vi "Save.vi"(7 "source paths":path[](array[path]), 8 "error in (no error)":errorcluster, 10 "processed sources":refnum<class "AB_Source.lvclass">[](array[class]), 11 "AB_EXE in":refnum<class "AB_EXE.lvclass">) -> (0 "error out":errorcluster, 1 "TypeInfo":string, 2 "source destination paths":path[](array[path]), 3 "AB_EXE out":refnum<class "AB_EXE.lvclass">, 4 "LEIFBuildData":u32, 5 "checksums":string[](array[string]))   [LabVIEW 2020, in "AB_EXE.lvclass"]
uses:
  <vilib>/AppBuilder/AB_Classes/EXE/AB_EXE.lvclass
  e:/builds/penguin/labview/branches/2020/dev/dist/vi.lib/AppBuilder/AB_Classes/TargetFile/AB_Targetfile.lvclass
  <vilib>/AppBuilder/AB_Classes/Source/AB_Source.lvclass
  <vilib>/AppBuilder/AB_Classes/Application/AB_Application.lvclass
  <vilib>/AppBuilder/AB_Classes/TargetFile/AB_Targetfile.lvclass
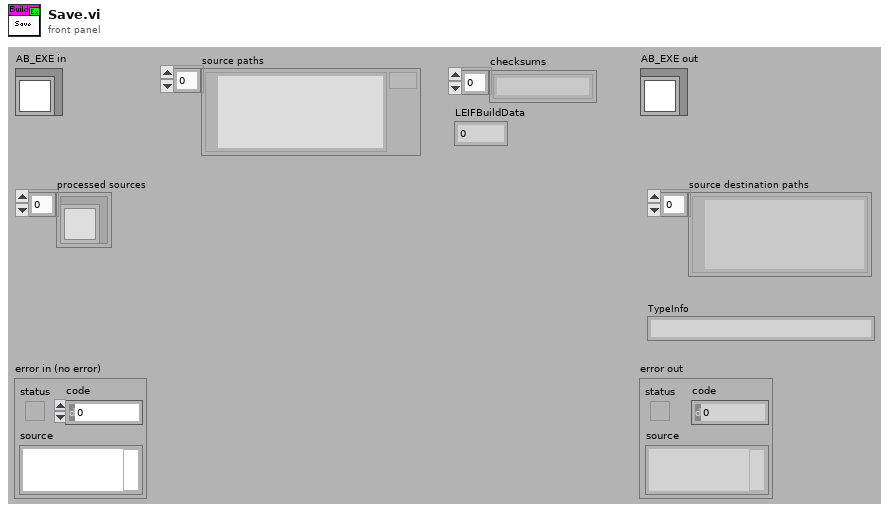
[diagram p1: front panel]
types:
  T1 = typedef "AB_Targetfile.ctl" = cluster{"targetfileName":string, "targetfileGUID":string, "enableDebugging":bool, "versionInfo":cluster{"productName":string, "legalCopyright":string, "companyName":string, "internalName":string, "fileDescription":string}, "eng_consolidatedTypeInfo":string, "fastFileFormat":bool, "eng_LEIFBuildData":u32, "versionIndependent":bool}
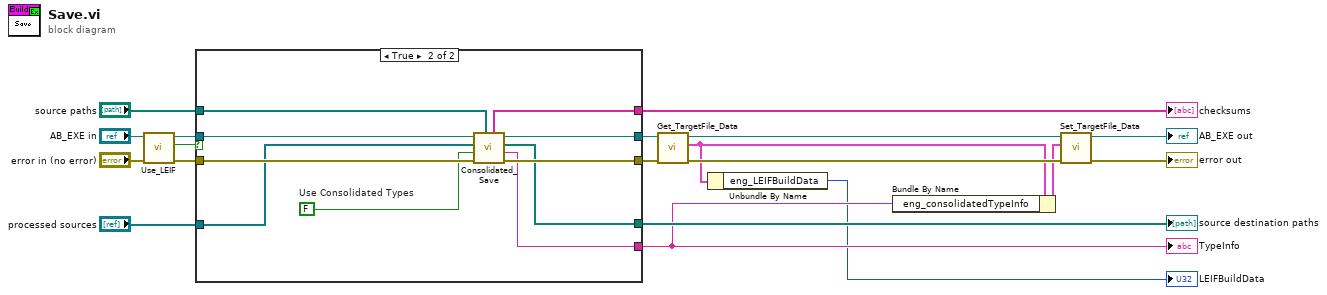
[diagram p0: block diagram]
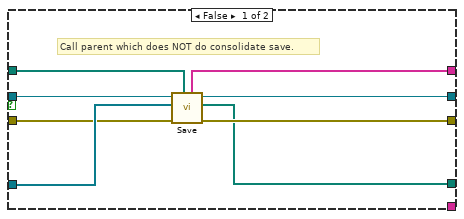
[diagram p2: hidden frame]
diagram:
  n1 = call <vilib>:"Use_LEIF.vi"("error in (no error)"="error in (no error)", "AB_Targetfile in"="AB_EXE in") -> ("error out"=w6:errorcluster, "use LEIF?"=w5:bool, "AB_Targetfile out"=w3:refnum<class "AB_EXE.lvclass">)  [unwired: 7 in]
  n2 = case shown="True" w5 {
    tunnel: "processed sources" -> [w23 w29]
    tunnel: w6 -> [w22 w30]
    tunnel: [w26 w36] -> w9
    tunnel: [w27 w35] -> w11
    tunnel: [_ w33] -> w8
    tunnel: "source paths" -> [w21 w31]
    tunnel: [w25 w34] -> w17
    tunnel: w3 -> [w24 w32]
    tunnel: [w20 w37] -> w16
    frame False {
      # "Call parent which does NOT do consolidate save."
      n3 = call-parent "Save.vi"("source paths"=w21, "error in"=w22, "processed sources"=w23, "AB_Build in"=w24) -> ("error out"=w26:errorcluster, "source destination paths"=w25:path[], "AB_Build out"=w27:refnum<class "AB_EXE.lvclass">, "checksums"=w20:string[])  [unwired: 2 in, 2 out]
    }
    frame True {
      w28 = FALSE  # Use Consolidated Types
      n4 = call <vilib>:"Consolidated_Save.vi"("source paths"=w31, "error in"=w30, "Use Consolidated Types"=w28, "processed sources"=w29, "AB_Targetfile in"=w32) -> ("error out"=w36:errorcluster, "TypeInfo"=w33:string, "source destination paths"=w34:path[], "AB_Targetfile out"=w35:refnum<class "AB_EXE.lvclass">, "checksums"=w37:string[])  [unwired: 2 in]
    }
  }
  "source destination paths" <- w17
  "TypeInfo" <- w8
  "checksums" <- w16
  n5 = call <vilib>:"Get_TargetFile_Data.vi"("error in (no error)"=w9, "AB_Targetfile in"=w11) -> ("error out"=w14:errorcluster, "data"=w2:T1, "AB_Targetfile out"=w15:refnum<class "AB_EXE.lvclass">)  [unwired: 7 in]
  n6 = Unbundle By Name(w2) -> ("eng_LEIFBuildData"=→"LEIFBuildData":u32)
  n7 = Bundle By Name(cluster=w2, "eng_consolidatedTypeInfo"=w8) -> (w13:T1)
  n8 = call <vilib>:"Set_TargetFile_Data.vi"("error in (no error)"=w14, "data"=w13, "AB_Targetfile in"=w15) -> ("error out"=→"error out":errorcluster, "AB_Targetfile out"=→"AB_EXE out":refnum<class "AB_EXE.lvclass">)  [unwired: 7 in]
